vi "Write Files.vi"(8 "error in (no error)":errorcluster, 11 "CHM Generator in":refnum<class "CHM Generator.lvclass">) -> (0 "error out":errorcluster, 3 "CHM Generator out":refnum<class "CHM Generator.lvclass">)   [LabVIEW 2020, in "CHM Generator.lvclass"]
uses:
  CHM Generator.lvclass
  CHM Generator.lvclass/CHM Generator.ctl
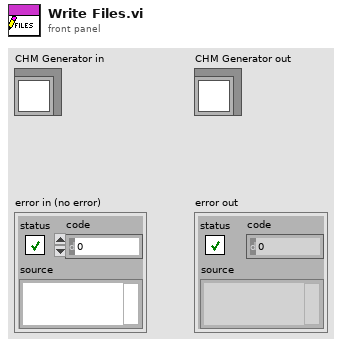
[diagram p1: front panel]
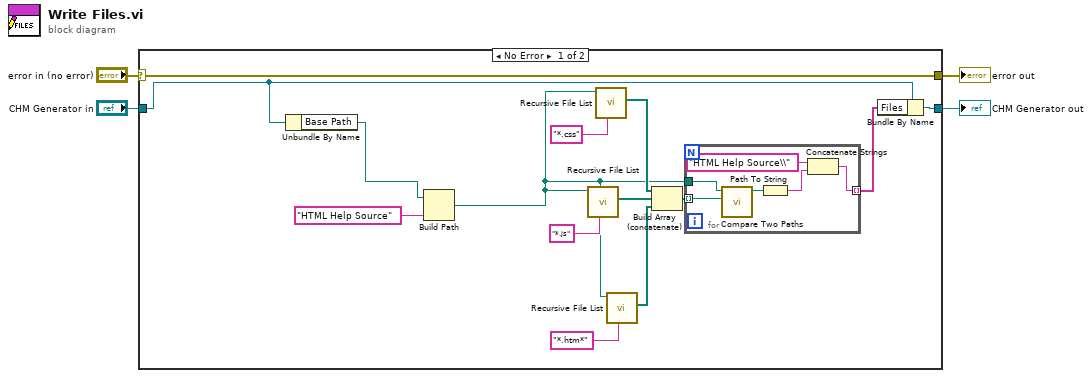
[diagram p0: block diagram]
diagram:
  n1 = case shown="No Error" "error in (no error)" {
    selector: "error in (no error)" -> [w18 w25]
    tunnel: [w18 w25] -> w3
    tunnel: [w17 w26] -> w1
    tunnel: "CHM Generator in" -> [w8 w26]
    frame No Error {
      n2 = Unbundle By Name(w8) -> ("Base Path"=w7:path)
      n3 = Build Path(base path=w7, name or relative path="HTML Help Source") -> (appended path=w6:path)
      n4 = call <vilib>:"Recursive File List.vi"("pattern"="*.js", "Folder Path"=w6) -> ("All Files in Dir"=w13:path[])  [unwired: 5 in, 4 out]
      n5 = call <vilib>:"Recursive File List.vi"("pattern"="*.css", "Folder Path"=w6) -> ("All Files in Dir"=w11:path[])  [unwired: 5 in, 4 out]
      n6 = call <vilib>:"Recursive File List.vi"("pattern"="*.htm*", "Folder Path"=w6) -> ("All Files in Dir"=w14:path[])  [unwired: 5 in, 4 out]
      n7 = Build Array (concatenate)(w11, w13, w14) -> (w10:path[])
      n8 = for {
        tunnel: w6 -> [w24]
        tunnel: w10 -> [w23] mode=indexing
        tunnel: [w19] -> w9 mode=indexing
        n9 = call <vilib>:"Compare Two Paths.vi"("Path 2"=w23, "Path 1"=w24) -> ("Relative Path from 1 to 2"=w22:path)  [unwired: 6 in, 3 out]
        n10 = Path To String(path=w22) -> (string=w20:string)
        n11 = Concatenate Strings("HTML Help Source\\" ("string"), w20) -> (w19:string)
      }
      n12 = Bundle By Name(cluster=w8, "Files"=w9) -> (w17:refnum<class "CHM Generator.lvclass">)
    }
    frame Error {
    }
  }
  "error out" <- w3
  "CHM Generator out" <- w1
